vi "GEA2 Collect HEWH ERDs.vi"(0 ".NET Refnum in":refnum<k24>, 1 "GEA Inputs":T3={"Source"=240, "Destination"=35} {"Destination" format="%.0x"; "Source" format="%.0x"}, 2 "GEA2 Event Registration In":refnum<event-registration>, 3 "Disable Electronic Mixing Valve (EMV) List":bool, 4 "Disable ERD (Main)":bool, 5 "error in (no error)":errorcluster, 6 "Custom ERDs":bool, 7 "Disable ERD Filter":bool, 8 "Retry Count":i32=5, 9 "#ERDs per message":i32=15, 10 "LV Program":T6, 12 "Read ERD List":T1[](array[typedef])=[{"ERD Number"=61623, "Data Type"=enum."string"}, {"ERD Number"=61617, "Data Type"=enum."string"}, {"ERD Number"=65314, "Data Type"=enum."string"}, {"ERD Number"=61563, "Data Type"=enum."string"}, {"ERD Number"=61537, "Data Type"=enum."uint32_t"}, {"ERD Number"=61612, "Data Type"=enum."string"}] {"ERD Number" format="%.0x"}, 13 "Enable Diagnostic Data":T4) -> (11 "ERD Data Out":T5[](array[typedef]) {"ERD Number" format="%.0x"}, 14 ".NET Refnum out":refnum<k24>, 15 "UnRead ERDs":i32, 16 "GEA2 Event Registration Out":refnum<event-registration>, 17 "ERD Array":string[][](array[string]), 19 "error out":errorcluster)   [LabVIEW 2016]
uses:
  C:/Technology Lab/NI-2010/Trunk/Utility/LabVIEW GEA2 Toolkit v1.0.0.0/Appliance.NET/GeaCommunication.dll
  Appliance.NET/GeaCommunication.dll
  type defs/Data Out.ctl
  Save File/File Setup (Public)/Type Definition/Save File DOE LabView Program.ctl
  type defs/ERD Read Data Out.ctl
  Washer HCC/Washer HCC NEWFI/Type Definitions/HCC Washer Types.ctl
  type defs/Source_Destination.ctl
  type defs/ERD Read Data In.ctl
  type defs/Data Type.ctl
  library/GEA2_Toolkit.lvlib
  Save File/File Setup.lvlib
panel:
  # "Core Location Setup"
  # "Output Data"
  # "Custom ERDs\n(Used for FP Motor\nController)"
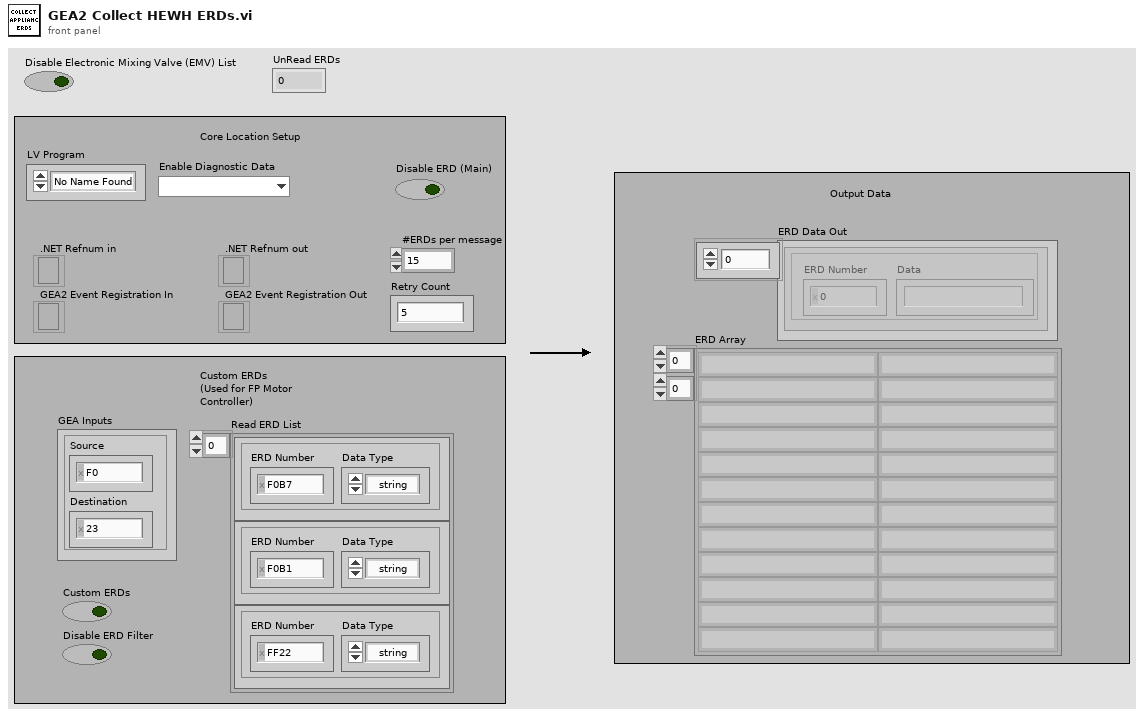
[diagram p1: front panel]
types:
  T1 = typedef "GEA2_Toolkit.lvlib/ERD Read Data In.ctl" = cluster{"ERD Number":u16, "Data Type":T2}
  T2 = typedef "GEA2_Toolkit.lvlib/Data Type.ctl" = enum16{"string", "boolean", "uint8_t", "uint16_t", "uint32_t", "uint64_t"}
  T3 = typedef "GEA2_Toolkit.lvlib/Source_Destination.ctl" = cluster{"Source":u8, "Destination":u8}
  T4 = typedef "HCC Washer Types.ctl" = enum16{"", "Viper Washer", "Hawk Washer", "2015 Washer", "2017 Washer"}
  T5 = typedef "GEA2_Toolkit.lvlib/ERD Read Data Out.ctl" = cluster{"ERD Number":u16, "Data":string}
  T6 = typedef "File Setup.lvlib/Save File DOE LabView Program.ctl" = enum16{"No Name Found", "DOE Stand", "Dishwasher Kitchen", "Portable Stand", "HEWH", "Dryer", "Dryer WILT", "HCC", "PRAT", "HEWH RLT", "Refrigeration"}
  T7 = typedef "HEWH ERD Data.ctl" = cluster{"ERD Therm Data":cluster{"T2":dbl, "T3a":dbl, "T3b":dbl, "T4":dbl, "T5":dbl, "T6":dbl, "Current":dbl, "Voltage":dbl, "EEV Possition":dbl, "Actual Set Point":dbl}, "ERD ENUM Data":cluster{"Actual Set Point":dbl, "Flow Events":string, "User Set Mode":string, "Operating Mode":string, "DRM Fallback Mode":string, "Vacation Fallback Mode":string, "User Set Point":dbl, "Vacation Set Point":dbl, "Vacation Remaining\n6":dbl}, "ERD DRM Data":cluster{"DRM Level":string, "DRM Override":string, "DRM Power":dbl, "DRM Energy":dbl}, "Fault Count":T8, "Relays":cluster{"DLB":bool, "Comp":bool, "UE":bool, "LE":bool, "Fan":bool}, "Comp Min On/Off Time":u16, "SS Run State":u16, "Condensate Drain Pan Voltage":u16, "CDP Triggered":bool, "Model Designator":u8, "Mixing Valve":T9}
  T8 = typedef "HEWH Faults.ctl" = cluster{"LE Fail":u32, "UE Fail":u32, "Comp Fail":u32, "T2 Fail":u32, "T3a Fail":u32, "T3b Fail":u32, "T4 Fail":u32, "T5 Fail":u32, "Cond A":u32, "Cond B":u32, "Cond C":u32, "Cond D":u32, "Cond E":u32, "Cond F":u32, "Cond G":u32, "Cond H":u32, "Cond I":u32, "Cond J":u32, "Cond L":u32, "Fan Fail":u32, "Dirty Filter":u32, "Dry Tank":u32}
  T9 = typedef "HEWH Mixing Valve.ctl" = cluster{"Tank Target Setpoint (0X4078)":dbl, "EMV Offset (0x4072)":dbl, "EMV Absolute Position (0x4073)":dbl, "Tank TCO State (0x4074)":string, "Outlet TCO State (0x4075)":string, "Fan PWM Drive %  (0x4076)":dbl, "FIRSTSTAGEKPQBITS (0x4079)":dbl, "FIRSTSTAGEKIQBITS (0x407A)":dbl, "FIRSTSTAGEKDQBITS (0x407B)":dbl, "SECONDSTAGEKPGAIN (0x408E)":dbl, "SECONDSTAGEKIGAIN (0x408F)":dbl, "SECONDSTAGEKDGAIN (0x4090)":dbl, "SECONDSTAGEKPQBITS (0x4091)":dbl, "SECONDSTAGEKIQBITS (0x4092)":dbl, "SECONDSTAGEKDQBITS (0x4093)":dbl, "THIRDSTAGEKPGAIN (0x4094)":dbl, "THIRDSTAGEKIGAIN (0x4095)":dbl, "THIRDSTAGEKDGAIN (0x4096)":dbl, "THIRDSTAGEKPQBITS (0x4097)":dbl, "THIRDSTAGEKIQBITS (0x4098)":dbl, "THIRDSTAGEKDQBITS (0x4099)":dbl, "FOURTHSTAGEKPGAIN (0x409A)":dbl, "FOURTHSTAGEKIGAIN (0x409B)":dbl, "FOURTHSTAGEKDGAIN (0x409C)":dbl, "FOURTHSTAGEKPQBITS (0x409D)":dbl, "FOURTHSTAGEKIQBITS (0x409E)":dbl, "FOURTHSTAGEKDQBITS (0x409F)":dbl, "MIXVALVEDELTAT (0x4077)":dbl, "PIDOUTPUTPOSITION (0x407C)":dbl, "T7 (0x407D)":dbl, "Cold Water Supply Temperature (0x40B7)":dbl, "Mixing Valve Flow State (0x407E)":string, "Mixing Valve PID Override (0x407F)":string}
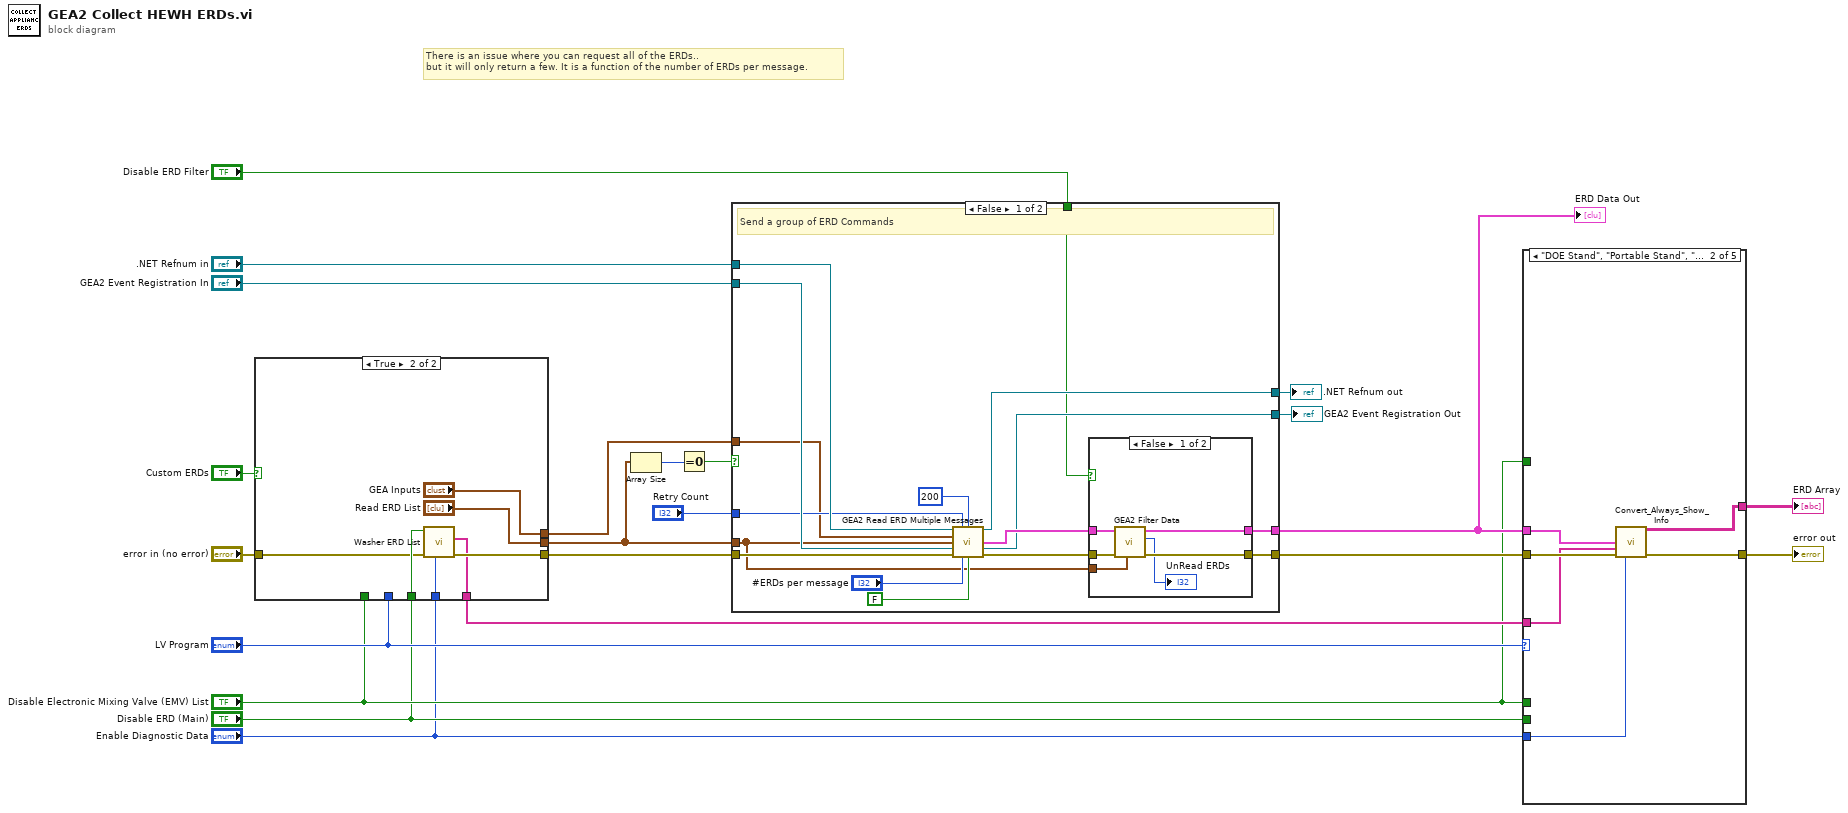
[diagram p0: block diagram]
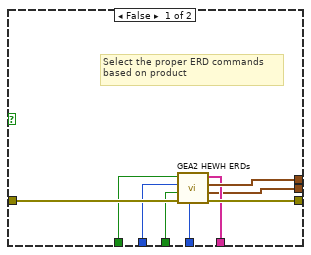
[diagram p2: hidden frame]
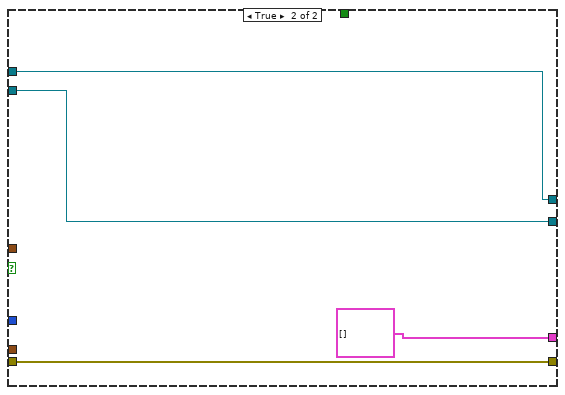
[diagram p4: hidden frame]
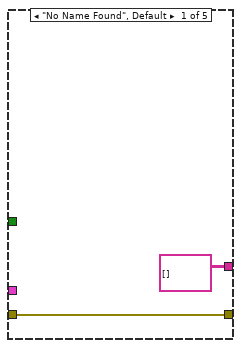
[diagram p5: hidden frame]
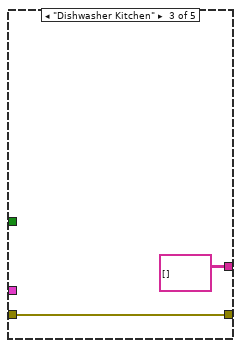
[diagram p6: hidden frame]
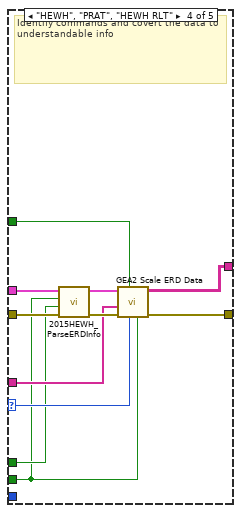
[diagram p7: hidden frame]
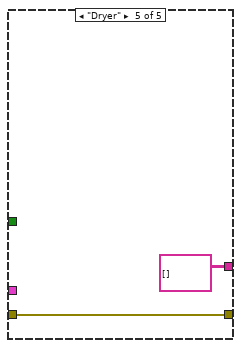
[diagram p8: hidden frame]
diagram:
  # "There is an issue where you can request all of the ERDs..\nbut it will only return a few. It is a function of the number of ERDs per message."
  n1 = case shown="True" "Custom ERDs" {
    tunnel: "error in (no error)" -> [w31 w34]
    tunnel: [w30 "GEA Inputs"] -> w21
    tunnel: [w29 w33] -> w20
    tunnel: "LV Program" -> [w28 _]
    tunnel: [w27 w32] -> w13
    tunnel: [w26 "Read ERD List"] -> w10
    tunnel: "Disable Electronic Mixing Valve (EMV) List" -> [w25 _]
    tunnel: "Disable ERD (Main)" -> [w24 w35]
    tunnel: "Enable Diagnostic Data" -> [w23 w36]
    frame False {
      # "Select the proper ERD commands \nbased on product"
      n2 = call "GEA2 HEWH ERDs.vi"("Enable Diagnostic Data"=w23, "Error In"=w31, "Disable ERD (Main)"=w24, "LV Program"=w28, "Disable Electronic Mixing Valve (EMV) List"=w25) -> ("Error Out"=w29:errorcluster, "Read ERD List"=w26:T1[], "GEA Inputs"=w30:T3, "ERD Headers"=w27:string[])  [unwired: 3 in]
    }
    frame True {
      n3 = call "Washer ERD List.vi"("Enable Diagnostic Data"=w36, "Error In"=w34, "Disable ERD (Main)"=w35) -> ("Error Out"=w33:errorcluster, "Header Array"=w32:string[])  [unwired: 6 in, 1 out]
    }
  }
  n4 = Array Size(array=w10) -> (size(s)=w9:i32)
  n5 = Equal To 0?(x=w9) -> (x = 0?=w8:bool)
  n6 = case shown="False" w8 {
    tunnel: w21 -> [w43 _]
    tunnel: w20 -> [w54 w66]
    tunnel: "GEA2 Event Registration In" -> [w53 w63]
    tunnel: ".NET Refnum in" -> [w52 w64]
    tunnel: "Retry Count" -> [w48 _]
    tunnel: [w46 T5[] [] ("ERD Data Out")] -> w16
    tunnel: [w44 w66] -> w11
    tunnel: w10 -> [w42 _]
    tunnel: [w41 w64] -> w6
    tunnel: [w40 w63] -> w5
    tunnel: "Disable ERD Filter" -> [w39 _]
    frame False {
      # "Send a group of ERD Commands"
      n7 = call "GEA2 Read ERD Multiple Messages.vi"("GEA2 Reference In"=w52, "Retry Count"=w48, "Read Timeout (ms)"=u32 200, "GEA Inputs"=w43, "Read ERD List"=w42, "GEA2 Event Registration"=w53, "Error In"=w54, "#ERDs per message"="#ERDs per message", "Verify ERD Response?"=FALSE) -> ("GEA2 Reference Out"=w41:refnum<k24>, "ERD Data Out"=w47:T5[], "Event Registration Refnum"=w40:refnum<event-registration>, "Error Out"=w45:errorcluster)  [unwired: 2 in, 1 out]
      n8 = case shown="False" w39 {
        tunnel: w47 -> [w60 w62]
        tunnel: [w59 w62] -> w46
        tunnel: w45 -> [w58 w61]
        tunnel: [w57 w61] -> w44
        tunnel: w42 -> [w56 _]
        frame False {
          n9 = call "GEA2 Filter Data.vi"("Read ERD List"=w56, "Error In"=w58, "ERD Data Out in"=w60) -> ("Error Out"=w57:errorcluster, "UnRead ERDs"=→"UnRead ERDs":i32, "ERD Data Out out"=w59:T5[])  [unwired: 6 in]
        }
        frame True {
        }
      }
    }
    frame True {
    }
  }
  "ERD Data Out" <- w16
  ".NET Refnum out" <- w6
  "GEA2 Event Registration Out" <- w5
  n10 = case shown="\"DOE Stand\", \"Portable Stand\", \"HCC\"" "LV Program" {
    selector: "LV Program" -> [_ _ _ w82 _]
    tunnel: w16 -> [_ w74 _ w87 _]
    tunnel: w11 -> [w67 w73 w75 w86 w89]
    tunnel: [w67 w72 w75 w84 w89] -> w14
    tunnel: w13 -> [_ w69 _ w81 _]
    tunnel: [string[][] [] ("ERD Array") w71 string[][] [] ("ERD Array") w83 string[][] [] ("ERD Array")] -> w12
    tunnel: "Disable Electronic Mixing Valve (EMV) List" -> [_ _ _ w79 _]
    tunnel: "Disable ERD (Main)" -> [_ _ _ w77 _]
    tunnel: "Disable Electronic Mixing Valve (EMV) List" -> [_ _ _ w78 _]
    tunnel: "Enable Diagnostic Data" -> [_ w70 _ _ _]
    frame "No Name Found", Default {
    }
    frame "DOE Stand", "Portable Stand", "HCC" {
      n11 = call "Convert_Always_Show_Info.vi"("Raw Data (ERD Input)"=w74, "ERD Headers"=w69, "Error In"=w73, "Enable Diagnostic Data"=w70) -> ("Data"=w71:string[][], "Error Out"=w72:errorcluster)  [unwired: 10 in]
    }
    frame "Dishwasher Kitchen" {
    }
    frame "HEWH", "PRAT", "HEWH RLT" {
      # "Identify commands and covert the data to understandable info"
      n12 = call "2015HEWH_ParseERDInfo.vi"("Error In"=w86, "Disable Electronic Mixing Valve (EMV) List"=w78, "Disable ERD (Main)"=w77, "ERD Data Out"=w87) -> ("Error Out"=w85:errorcluster, "ERD Data"=w80:T7)  [unwired: 6 in]
      n13 = call "GEA2 Scale ERD Data.vi"("Disable ERD (Main)"=w77, "LV Program"=w82, "Disable Electronic Mixing Valve (EMV) List"=w79, "Error In"=w85, "Headers"=w81, "HEWH ERD Data"=w80) -> ("Error Out"=w84:errorcluster, "ERD Array"=w83:string[][])  [unwired: 4 in]
    }
    frame "Dryer" {
    }
  }
  "ERD Array" <- w12
  "error out" <- w14
